vi "niFpgaDeadZoneTemplate.vi"(0 "start of dead zone":fxp<+/-,16,16>, 5 "input":fxp<+/-,16,16>, 9 "end of dead zone":fxp<+/-,16,16> format="%04x") -> (4 "output":fxp<+/-,16,16>)   [LabVIEW 2017]
doc: "Provides a region of zero output, or a dead zone. <B>output</B> is zero if <B>start of dead zone</B> <= <B>input</B> <= <B>end of dead zone</B>. The data type you wire to <B>input</B> determines the <B>output</B> data type."
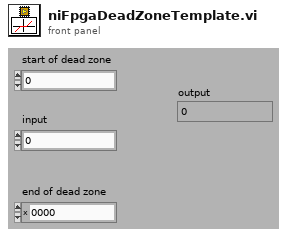
[diagram p1: front panel]
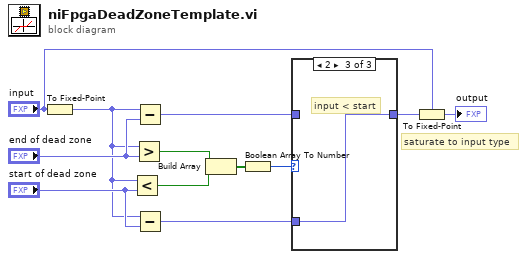
[diagram p0: block diagram]
diagram:
  # "saturate to input type"
  n1 = To Fixed-Point(number="input") -> (fixed-point=w4:fxp<+/-,16,16>)  [unwired: 1 in]
  n2 = Less?(x=w4, y="start of dead zone") -> (x < y?=w9:bool)
  n3 = Greater?(x=w4, y="end of dead zone") -> (0:w10:bool)
  n4 = Subtract(x=w4, y="end of dead zone") -> (x-y=w2:fxp<+/-,17,17>)
  n5 = Subtract(x=w4, y="start of dead zone") -> (x-y=w1:fxp<+/-,17,17>)
  n6 = Build Array(w10, w9) -> (w12:bool[])
  n7 = Boolean Array To Number(Boolean array=w12) -> (number=w11:u8)
  n8 = case shown="2" w11 {
    tunnel: [_ w13 w14] -> w6
    tunnel: w2 -> [_ w13 _]
    tunnel: w1 -> [_ _ w14]
    frame 0, Default {
      # "in dead zone"
    }
    frame 1 {
      # "input > end"
    }
    frame 2 {
      # "input < start"
    }
  }
  n9 = To Fixed-Point(fixed-point type="input", number=w6) -> (fixed-point=→"output":fxp<+/-,16,16>)
